vi "Insert Element.vi"(8 "error in (no error)":errorcluster, 9 "Value":bool, 10 "Insert Index":i32, 11 "Array1D_Bool in":refnum<class "Array1D_Bool.lvclass">) -> (0 "error out":errorcluster, 3 "Array1D_Bool out":refnum<class "Array1D_Bool.lvclass">)   [LabVIEW 2021, in "Array1D_Bool.lvclass"]
uses:
  Array1D_Bool.lvclass
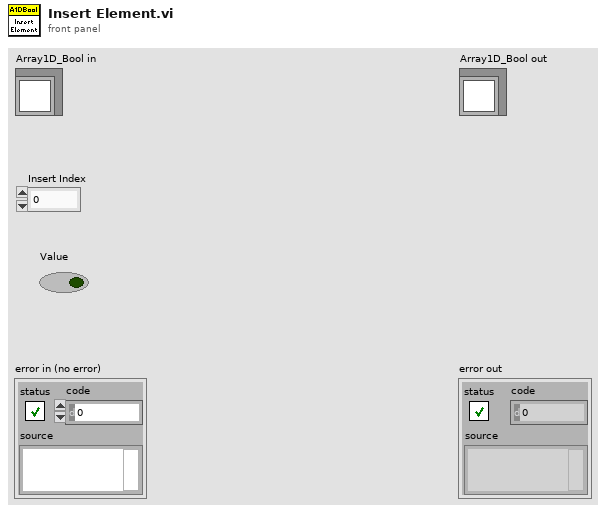
[diagram p1: front panel]
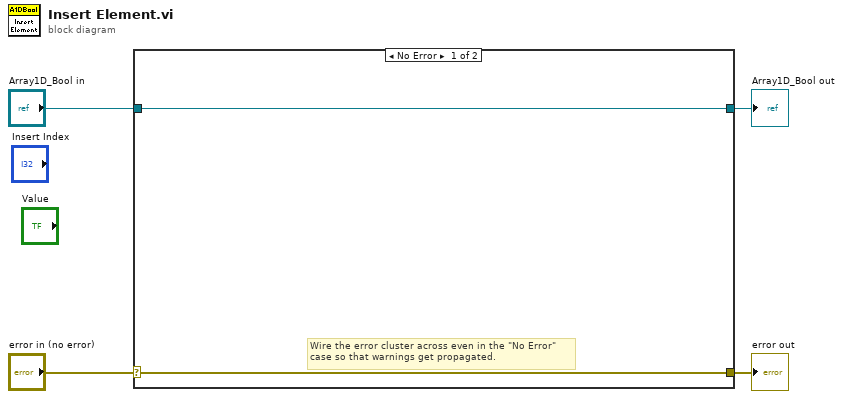
[diagram p0: block diagram]
diagram:
  n1 = case shown="No Error" "error in (no error)" {
    selector: "error in (no error)" -> [w5 w8]
    tunnel: [w5 w8] -> w3
    tunnel: [w6 w7] -> w1
    tunnel: "Array1D_Bool in" -> [w6 w7]
    frame No Error {
      # "Wire the error cluster across even in the \"No Error\"\ncase so that warnings get propagated."
    }
    frame Error {
    }
  }
  "error out" <- w3
  "Array1D_Bool out" <- w1
